vi "hidden_deltas(b).vi"(9 "Forward Delta":dbl[](array[numeric]), 10 "Forward Biases":dbl[](array[numeric]), 11 "Node Outputs":dbl[](array[numeric])) -> (3 "Current Delta":dbl[](array[numeric]))   [LabVIEW 2018]
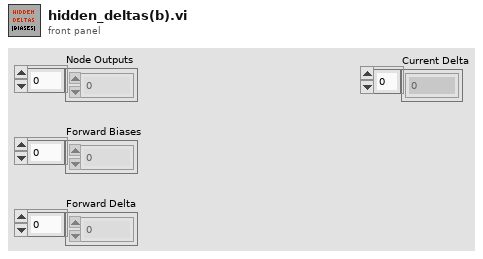
[diagram p1: front panel]
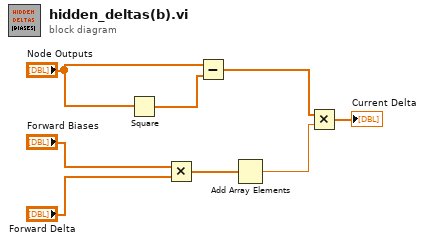
[diagram p0: block diagram]
diagram:
  n1 = Square(x="Node Outputs") -> (x^2=w5:dbl[])
  n2 = Multiply(x="Forward Biases", y="Forward Delta") -> (x*y=w4:dbl[])
  n3 = Subtract(x="Node Outputs", y=w5) -> (x-y=w3:dbl[])
  n4 = Add Array Elements(numeric array=w4) -> (sum=w2:dbl)
  n5 = Multiply(x=w3, y=w2) -> (x*y=→"Current Delta":dbl[])
